vi "SetParam.vi"(8 "error in (no error)":errorcluster caption="entrée d'erreur (pas d'erreur)", 10 "RBFSampler":T1={"gamma"=1.0, "n_components"=100, "random_state"=-1} {"random_state" min=-1}, 11 "RBFSampler.lvclass":refnum<class "RBFSampler.lvclass">) -> (0 "error out":errorcluster caption="sortie d'erreur", 3 "RBFSampler.lvclass":refnum<class "RBFSampler.lvclass">)   [LabVIEW 2020, in "RBFSampler.lvclass"]
doc: "Set Parameters"
uses:
  RBFSampler.lvclass
  RBFSampler.lvclass/RBFSampler.ctl
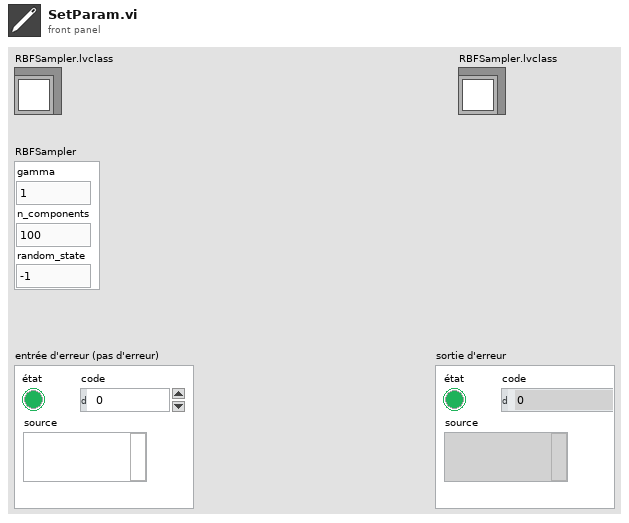
[diagram p1: front panel]
types:
  T1 = cluster{"gamma":dbl, "n_components":i32, "random_state":i32}
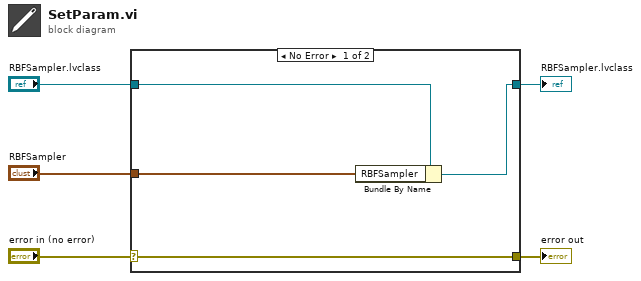
[diagram p0: block diagram]
diagram:
  n1 = case shown="No Error" "error in (no error)" {
    selector: "error in (no error)" -> [w9 w10]
    tunnel: [w9 w10] -> w4
    tunnel: [w7 w11] -> w2
    tunnel: "RBFSampler.lvclass" -> [w8 w11]
    tunnel: "RBFSampler" -> [w6 _]
    frame No Error {
      n2 = Bundle By Name(cluster=w8, "RBFSampler"=w6) -> (w7:refnum<class "RBFSampler.lvclass">)
    }
    frame Error {
    }
  }
  "error out" <- w4
  "RBFSampler.lvclass" <- w2
